vi "readLogAppliedSettingsMatchStart.vi"(8 "error in (no error)":errorcluster, 10 "Parser":refnum<class "U8ArrayParserAutoIndexing.lvclass">, 11 "M1M3SAL in":refnum<class "M1M3SAL.lvclass">) -> (0 "error out":errorcluster, 2 "EventAppliedSettingsMatchStart":variant, 3 "M1M3SAL out":refnum<class "M1M3SAL.lvclass">)   [LabVIEW 2016, in "M1M3SupportCommunicator.lvlib" / "M1M3SAL.lvclass"]
uses:
  M1M3SAL.lvclass
  Common_RT_Utilities/U8ArrayParserAutoIndexing/U8ArrayParserAutoIndexing.lvclass
  DataTypes/Topics/EventAppliedSettingsMatchStart.ctl
  DataTypes/Topics/Parts/Timestamp.ctl
  DataTypes/Topics/M1M3SupportTopics.lvlib
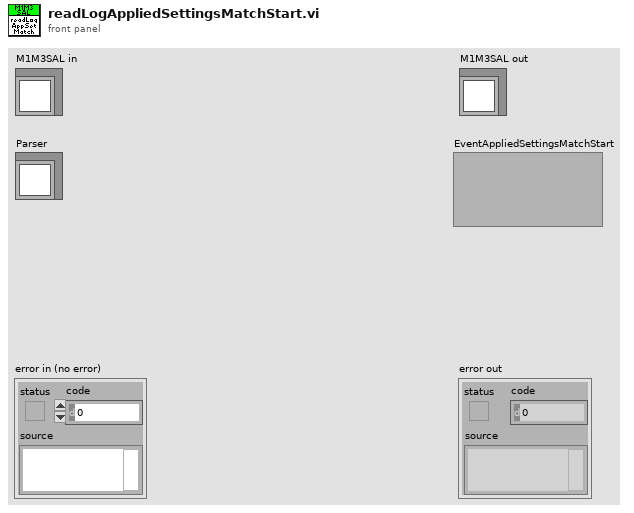
[diagram p1: front panel]
types:
  T1 = typedef "M1M3SupportTopics.lvlib/EventAppliedSettingsMatchStart.ctl" = cluster{"Timestamp":T2, "AppliedSettingsMatchStart":bool}
  T2 = typedef "M1M3SupportTopics.lvlib/Timestamp.ctl" = dbl
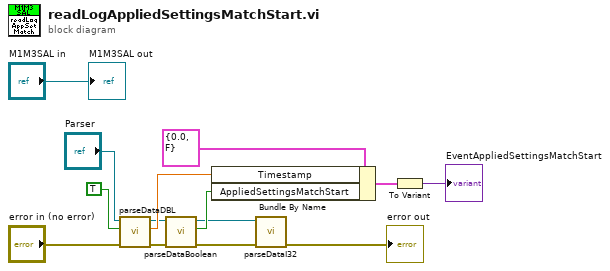
[diagram p0: block diagram]
diagram:
  n1 = call "parseDataDBL.vi"("error in (no error)"="error in (no error)", "OverrideSwapBytes"=TRUE, "U8ArrayParserAutoIndexing in"="Parser") -> ("error out"=w2:errorcluster, "Data"=w7:dbl, "U8ArrayParserAutoIndexing out"=w6:refnum<class "U8ArrayParserAutoIndexing.lvclass">)  [unwired: 6 in]
  n2 = call "parseDataBoolean.vi"("error in (no error)"=w2, "U8ArrayParserAutoIndexing in"=w6) -> ("error out"=w3:errorcluster, "Data"=w5:bool, "U8ArrayParserAutoIndexing out"=w4:refnum<class "U8ArrayParserAutoIndexing.lvclass">)  [unwired: 7 in]
  n3 = Bundle By Name(cluster=T1 {"Timestamp"=0.0, "AppliedSettingsMatchStart"=FALSE} ("EventAppliedSettingsMatchStart"), "Timestamp"=w7, "AppliedSettingsMatchStart"=w5) -> (w13:T1)
  n4 = call "parseDataI32.vi"("error in (no error)"=w3, "U8ArrayParserAutoIndexing in"=w4) -> ("error out"=→"error out":errorcluster)  [unwired: 7 in, 2 out]
  n5 = To Variant(anything=w13) -> (Variant=→"EventAppliedSettingsMatchStart":variant)
  "M1M3SAL out" <- "M1M3SAL in"
